vi "System_Data_Load.vi"(8 "error in":errorcluster) -> (0 "error out":errorcluster, 3 "System Data":T1={"System"={"Active"=FALSE, "Exit"=FALSE, "Command wait"="", "Status_Time"=0, "Time_GPS"=0}, "Stepper Motor"={"Connection Reference"="", "Valid Connection"=FALSE, "Speed"=15}, "Camera Data"={"Image path"=path "", "Filenames"=[], "Filenames queue"=[]}, "Core"={"Close Panel on Exit?"=FALSE, "Current VI Reference"=refnum}} {"Stepper Motor"."Speed" scale=0.0..30.0})   [LabVIEW 2019]
uses:
  System Data.ctl
  Stepper Data.ctl
  Camera Data.ctl
  <vilib>/Utility/xml.llb/Read From XML File(string).vi
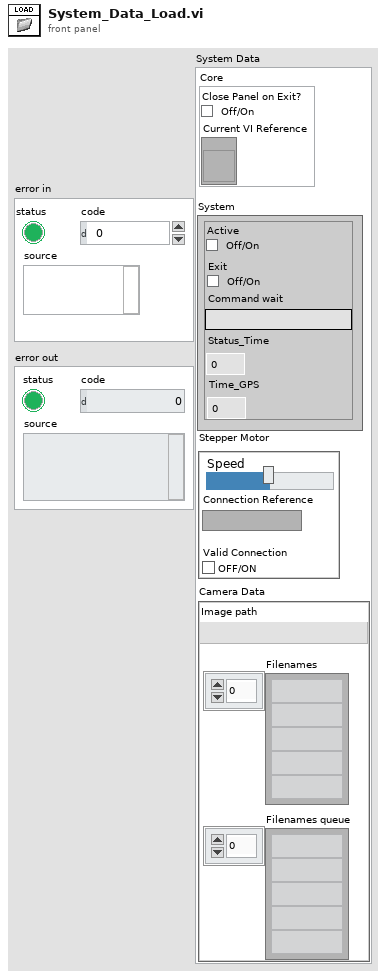
[diagram p1: front panel]
types:
  T1 = typedef "System Data.ctl" = cluster{"System":cluster{"Active":bool, "Exit":bool, "Command wait":string, "Status_Time":i32, "Time_GPS":i32}, "Stepper Motor":T2, "Camera Data":T3, "Core":cluster{"Close Panel on Exit?":bool, "Current VI Reference":refnum<vi>}}
  T2 = typedef "Stepper Data.ctl" = cluster{"Connection Reference":refnum<visa-resource-name>, "Valid Connection":bool, "Speed":i32}
  T3 = typedef "Camera Data.ctl" = cluster{"Image path":path, "Filenames":string[], "Filenames queue":string[]}
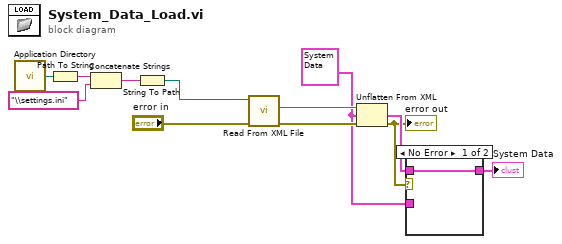
[diagram p0: block diagram]
diagram:
  w2 = T1 {"System"={"Active"=FALSE, "Exit"=FALSE, "Command wait"="", "Status_Time"=0, "Time_GPS"=0}, "Stepper Motor"={"Connection Reference"="", "Valid Connection"=FALSE, "Speed"=15}, "Camera Data"={"Image path"=path "", "Filenames"=[], "Filenames queue"=[]}, "Core"={"Close Panel on Exit?"=FALSE, "Current VI Reference"=refnum}} ("System Data")
  n1 = call <vilib>:"Application Directory.vi"() -> ("Application Directory"=w11:path)
  n2 = Path To String(path=w11) -> (string=w12:string)
  n3 = Concatenate Strings(w12, "\\settings.ini" ("string")) -> (w9:string)
  n4 = String To Path(string=w9) -> (path=w7:path)
  n5 = call-poly <vilib>:"Read From XML File.vi"("error in (no error)"="error in", "XML File Path"=w7) -> ("error out"=w5:errorcluster, "XML Elements"=w6:string)  [unwired: 7 in, 1 out]
  n6 = Unflatten From XML(xml string=w6, type=w2, error in (no error)=w5) -> (value=w4:T1, error out=w3:errorcluster)
  "error out" <- w3
  n7 = case shown="No Error" w3 {
    tunnel: [w13 w14] -> w1
    tunnel: w2 -> [_ w14]
    tunnel: w4 -> [w13 _]
    frame No Error {
    }
    frame Error {
    }
  }
  "System Data" <- w1
